vi "Obtain Command Event.vi"(0 "Local Listener Session":T1, 11 "error in (no error)":errorcluster) -> (6 "REx Template Event":refnum<user-event>, 15 "error out":errorcluster)   [LabVIEW 2012, in "REx.lvlib" / "REx - CMD_TEMPLATE.lvclass"]
uses:
  REx - CMD_TEMPLATE.lvclass
  _REx/Components/Local Listener Session/Typedefs/Session Handle.ctl
  _REx/Components/Local Listener Session/Local Listener Session.lvclass
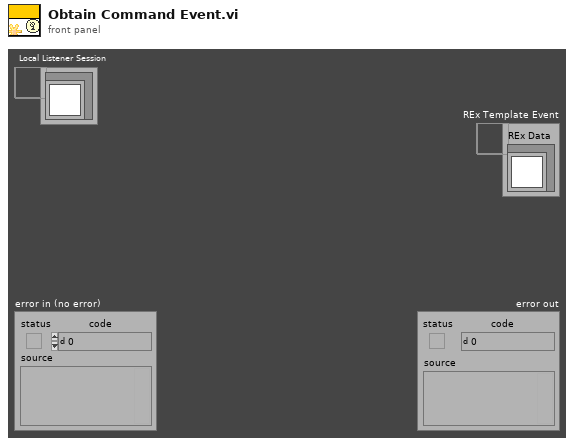
[diagram p1: front panel]
types:
  T1 = typedef "REx.lvlib/Local Listener Session.lvclass/Session Handle.ctl" = refnum<data-value>
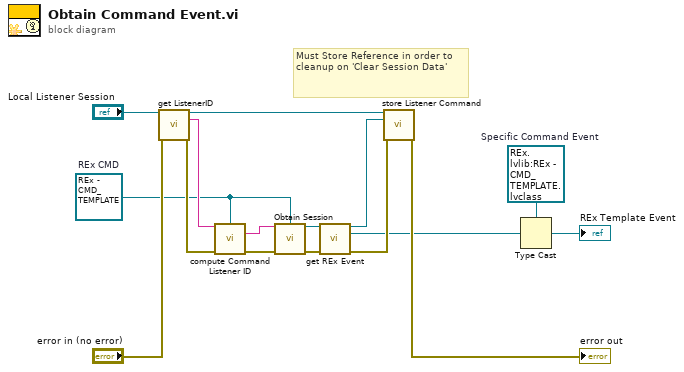
[diagram p0: block diagram]
diagram:
  w12 = refnum<user-event> refnum  # Specific Command Event
  w6 = refnum<class "REx - CMD_TEMPLATE.lvclass"> refnum  # REx CMD
  # "Must Store Reference in order to cleanup on 'Clear Session Data'"
  n1 = call "get ListenerID.vi"("Session Handle in"="Local Listener Session", "error in (no error)"="error in (no error)") -> ("Session Handle out"=w5:T1, "Session Name"=w15:string, "error out"=w16:errorcluster)  [unwired: 11 in]
  n2 = call-dynamic "compute Command Listener ID.vi"("Listener Session ID"=w15, "REx - Command ROOT"=w6, "error in"=w16) -> ("Command Listener ID"=w7:string, "error out"=w9:errorcluster)  [unwired: 11 in]
  n3 = call "Obtain Session.vi"("Listener ID ()"=w7, "REx Command"=w6, "error in (no error)"=w9) -> ("Listener Session Handle"=w14:T1, "error out"=w13:errorcluster)  [unwired: 9 in, 2 out]
  n4 = call "get REx Event.vi"("Session Handle in"=w14, "error in (no error)"=w13) -> ("Session Handle out"=w1:T1, "Command Event"=w2:refnum<user-event>, "error out"=w4:errorcluster)  [unwired: 11 in]
  n5 = call "store Listener Command.vi"("Listener Handle in"=w5, "Command Handle in"=w1, "error in (no error)"=w4) -> ("error out"=→"error out":errorcluster)  [unwired: 11 in, 1 out]
  n6 = Type Cast(type=w12, x=w2) -> (*(type *) &x=→"REx Template Event":refnum<user-event>)
